vi "Autonomous Independent.vi"   [LabVIEW 2013]
doc: "This VI is called when autonomous begins, and will automatically be terminated when autonomous ends. You can carry out timed or sensor driven robot movement independently without needing to return to the caller."
uses:
  <vilib>/Rock Robotics/WPI/Solenoid/WPI_SolenoidValue.ctl
  Robot Global Data.vi
  <vilib>/Rock Robotics/WPI/RobotDrive/WPI_RobotDriveGetSetRefNum.vi
  <vilib>/Rock Robotics/WPI/RobotDrive/WPI_RobotDriveArcadeDrive_Standard(NoSaturation).vi
  <vilib>/Rock Robotics/WPI/Solenoid/WPI_SolenoidSetEnum.vi
panel:
  # "Be sure to right-click and choose Data Operations>>Make Current Value default if you want to save the array values with the VI"
types:
  T1 = typedef "WPI_RobotDriveDevRef.ctl" = cluster{"DevStatus":errorcluster, "Motors[]":T2[], "Square Inputs":bool, "Max Output":dbl, "Isochronous":bool}
  T2 = typedef "WPI_MotorControlDeviceRef.ctl" = cluster{"DeviceStatus":errorcluster, "Type":enum16{"PWM", "CAN"}, "PWM":cluster{"Digital Module":T3, "PWM Channel":T4, "DeadBand":T5}, "CAN":cluster{"Device Number":u8, "Control Mode":T6, "Semaphore":T7, "Max Vout":dbl}, "Invert":bool, "TransformRef":T8, "InvTransformRef":T8}
  T3 = typedef "FPGA_TypedefDigitalModule.ctl" = enum16{"Digital Module 1", "Digital Module 2"}
  T4 = typedef "FPGA_DIOPWMChannel.ctl" = enum8{"PWM 1", "PWM 2", "PWM 3", "PWM 4", "PWM 5", "PWM 6", "PWM 7", "PWM 8", "PWM 9", "PWM 10", "Invalid"}
  T5 = typedef "WPI_PWMDeadband.ctl" = cluster{"Name":string, "maxPositivePwm":i32, "minPositivePwm":i32, "centerPwm":i32, "maxNegativePwm":i32, "minNegativePwm":i32, "angularRange":u16}
  T6 = typedef "WPI_CANJaguar_ControlMode.ctl" = enum8{"Percent VBus", "Current", "Speed", "Position", "Voltage"}
  T7 = typedef "Semaphore RefNum" = refnum<k1>
  T8 = typedef "WPI_PWMTransform_ConPane.ctl" = refnum<vi>
  T9 = typedef "WPI_SolenoidValue.ctl" = enum16{"Off", "On", "Forward", "Reverse"}
  T10 = typedef "WPI_DigitalInputDevRef.ctl" = cluster{"DevStatus":errorcluster, "DIO Channel":T11, "Digital Module":T3}
  T11 = typedef "FPGA_DIOChannel.ctl" = enum8{"DIO 1", "DIO 2", "DIO 3", "DIO 4", "DIO 5", "DIO 6", "DIO 7", "DIO 8", "DIO 9", "DIO 10", "DIO 11", "DIO 12", "DIO 13", "DIO 14", "Invalid"}
  T12 = typedef "WPI_SolenoidDevRef.ctl" = cluster{"DevStatus":errorcluster, "Solenoid Module":T13, "Forward Solenoid Channel":T14, "Reverse Solenoid Channel":T14}
  T13 = typedef "FPGA_TypedefSolenoidModule.ctl" = enum16{"Solenoid Module 1", "Solenoid Module 2"}
  T14 = typedef "WPI_SolenoidChannel.ctl" = enum8{"Solenoid 1", "Solenoid 2", "Solenoid 3", "Solenoid 4", "Solenoid 5", "Solenoid 6", "Solenoid 7", "Solenoid 8", "Invalid"}
  T15 = typedef "WPI_AnalogChannelDevRef.ctl" = cluster{"DevStatus":errorcluster, "Analog Module":T16, "Analog Channel":T17}
  T16 = typedef "FPGA_TypedefAnalogModule.ctl" = enum16{"Analog Module 1", "Analog Module 2"}
  T17 = typedef "FPGA_AIChannel.ctl" = enum8{"AI 1", "AI 2", "AI 3", "AI 4", "AI 5", "AI 6", "AI 7", "AI 8", "Invalid"}
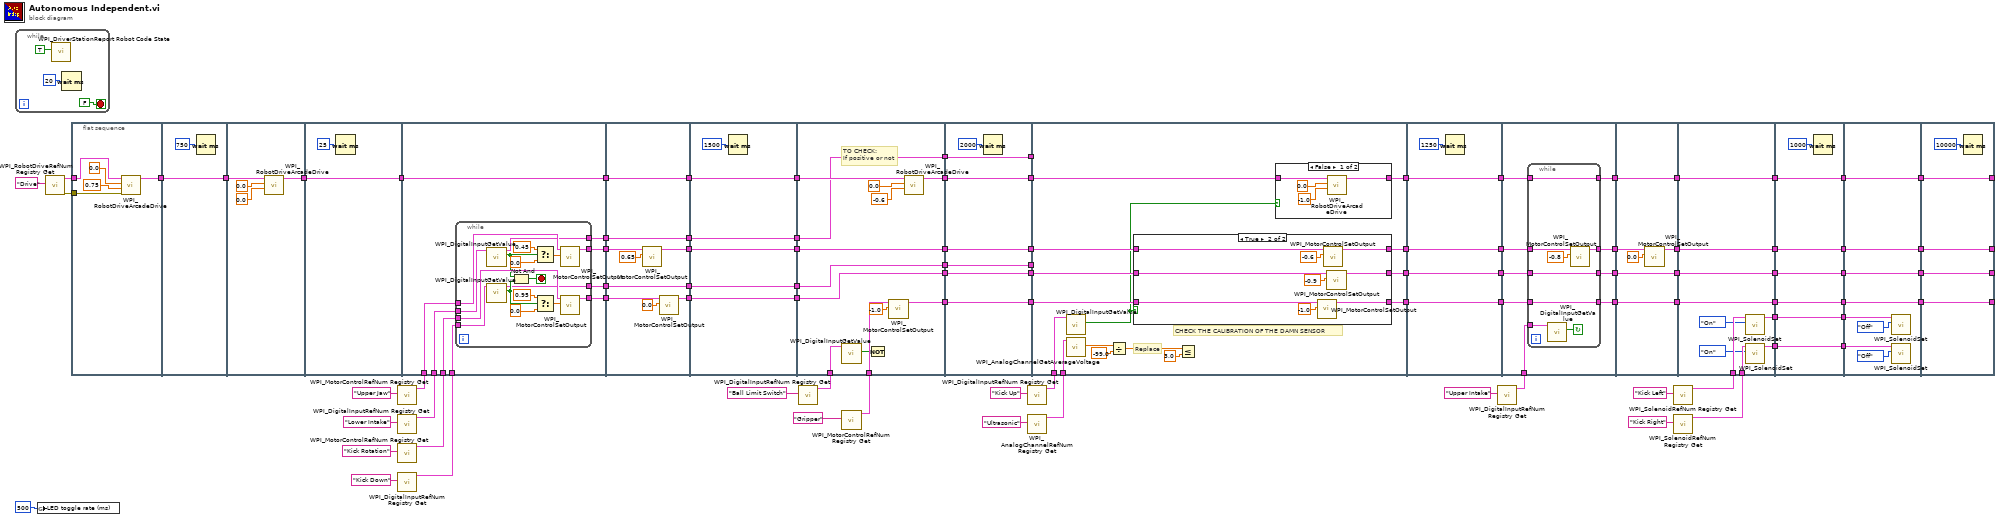
[diagram p0: block diagram]
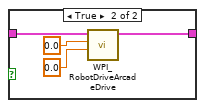
[diagram p2: hidden frame]
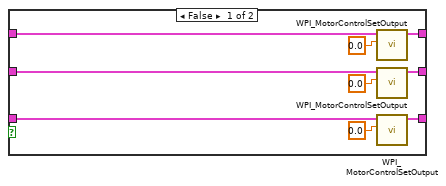
[diagram p3: hidden frame]
diagram:
  n1 = while {
    stop <- FALSE stop-if-true
    n2 = call <vilib>:"WPI_DriverStationReport Robot Code State.vi"("Autonomous"=TRUE) -> ()  [unwired: 10 in, 1 out]
    n3 = Wait (ms)(milliseconds to wait=u32 20) -> ()  [unwired: 1 out]
  }
  n4 = global write "Robot Global Data.vi" "LED toggle rate (ms)"(u32 500 ("LED ms toggle rate")) -> ()
  n5 = call <vilib>:"WPI_RobotDriveRefNum Registry Get.vi"("refnum name"="Drive") -> ("error out"=w84:errorcluster, "RobotDriveDevRef"=w85:T1)  [unwired: 9 in]
  n6 = flat-sequence {
    tunnel: w85 -> [w95]
    tunnel: w84 -> [w94]
    tunnel: [w93] -> w73
    tunnel: w73 -> [w99]
    tunnel: [w99] -> w72
    tunnel: [w102] -> w71
    tunnel: w72 -> [w103]
    tunnel: w71 -> [w105]
    tunnel: [w105] -> w70
    tunnel: w83 -> [w113]
    tunnel: w81 -> [w110]
    tunnel: w78 -> [w114]
    tunnel: [w112] -> w77
    tunnel: w70 -> [w112]
    tunnel: w76 -> [w111]
    tunnel: [w109] -> w75
    tunnel: [w108] -> w74
    tunnel: [w107] -> w69
    tunnel: [w106] -> w68
    tunnel: w77 -> [w136]
    tunnel: w75 -> [w139]
    tunnel: w74 -> [w140]
    tunnel: w69 -> [w133]
    tunnel: w68 -> [w135]
    tunnel: [w136] -> w10
    tunnel: [w135] -> w8
    tunnel: [w134] -> w6
    tunnel: [w133] -> w4
    tunnel: [w132] -> w2
    tunnel: w10 -> [w146]
    tunnel: [w146] -> w9
    tunnel: w8 -> [w145]
    tunnel: [w145] -> w7
    tunnel: w6 -> [w144]
    tunnel: [w144] -> w5
    tunnel: w4 -> [w143]
    tunnel: [w143] -> w3
    tunnel: w2 -> [w142]
    tunnel: [w142] -> w1
    tunnel: w9 -> [w159]
    tunnel: w67 -> [w158]
    tunnel: [w157] -> w22
    tunnel: [w156] -> w20
    tunnel: w65 -> [w155]
    tunnel: [w154] -> w18
    tunnel: w7 -> [w154]
    tunnel: [w153] -> w16
    tunnel: w5 -> [w153]
    tunnel: [w152] -> w14
    tunnel: w3 -> [w152]
    tunnel: [w151] -> w12
    tunnel: w1 -> [w151]
    tunnel: w22 -> [w166]
    tunnel: [w166] -> w21
    tunnel: w20 -> [w165]
    tunnel: [w165] -> w19
    tunnel: w18 -> [w164]
    tunnel: [w164] -> w17
    tunnel: w16 -> [w163]
    tunnel: [w163] -> w15
    tunnel: w14 -> [w162]
    tunnel: [w162] -> w13
    tunnel: w12 -> [w161]
    tunnel: [w161] -> w11
    tunnel: w21 -> [w181]
    tunnel: w19 -> [w178]
    tunnel: w17 -> [_]
    tunnel: w15 -> [w179]
    tunnel: w13 -> [_]
    tunnel: w11 -> [w177]
    tunnel: w63 -> [w180]
    tunnel: w61 -> [w176]
    tunnel: [w175] -> w30
    tunnel: [w174] -> w28
    tunnel: [w173] -> w26
    tunnel: [w172] -> w24
    tunnel: w30 -> [w212]
    tunnel: [w212] -> w29
    tunnel: w28 -> [w211]
    tunnel: [w211] -> w27
    tunnel: w26 -> [w210]
    tunnel: [w210] -> w25
    tunnel: w24 -> [w209]
    tunnel: [w209] -> w23
    tunnel: w29 -> [w221]
    tunnel: w27 -> [w219]
    tunnel: w59 -> [w218]
    tunnel: w25 -> [w215]
    tunnel: w23 -> [w213]
    tunnel: [w220] -> w58
    tunnel: [w217] -> w57
    tunnel: [w216] -> w56
    tunnel: [w214] -> w55
    tunnel: w58 -> [w235]
    tunnel: w57 -> [w232]
    tunnel: w56 -> [w234]
    tunnel: w55 -> [w233]
    tunnel: [w235] -> w54
    tunnel: [w234] -> w53
    tunnel: [w233] -> w52
    tunnel: [w230] -> w51
    tunnel: w54 -> [w245]
    tunnel: w53 -> [w244]
    tunnel: w52 -> [w243]
    tunnel: w51 -> [w242]
    tunnel: w48 -> [w241]
    tunnel: w47 -> [w240]
    tunnel: [w245] -> w46
    tunnel: [w244] -> w44
    tunnel: [w243] -> w42
    tunnel: [w242] -> w40
    tunnel: [w237] -> w38
    tunnel: [w236] -> w36
    tunnel: w46 -> [w252]
    tunnel: [w252] -> w45
    tunnel: w44 -> [w251]
    tunnel: [w251] -> w43
    tunnel: w42 -> [w250]
    tunnel: [w250] -> w41
    tunnel: w40 -> [w249]
    tunnel: [w249] -> w39
    tunnel: w38 -> [w248]
    tunnel: [w248] -> w37
    tunnel: w36 -> [w247]
    tunnel: [w247] -> w35
    tunnel: w45 -> [w260]
    tunnel: w43 -> [w259]
    tunnel: w41 -> [w258]
    tunnel: w39 -> [w257]
    tunnel: w37 -> [w255]
    tunnel: w35 -> [w256]
    tunnel: [w260] -> w34
    tunnel: [w259] -> w33
    tunnel: [w258] -> w32
    tunnel: [w257] -> w31
    tunnel: [w262] -> _
    tunnel: [w263] -> _
    tunnel: [w264] -> _
    tunnel: [w265] -> _
    tunnel: w34 -> [w265]
    tunnel: w33 -> [w264]
    tunnel: w32 -> [w263]
    tunnel: w31 -> [w262]
    frame #0 {
      n7 = call-poly <vilib>:"WPI_RobotDriveArcadeDrive.vi"("error in (no error)"=w94, "Y axis value"=0.75, "X axis value"=0.0, "RobotDriveDevRef"=w95) -> ("RobotDriveDevRef"=w93:T1)  [unwired: 5 in, 2 out]
    }
    frame #1 {
      n8 = Wait (ms)(milliseconds to wait=u32 750) -> ()  [unwired: 1 out]
    }
    frame #2 {
      n9 = call-poly <vilib>:"WPI_RobotDriveArcadeDrive.vi"("Y axis value"=0.0, "X axis value"=0.0, "RobotDriveDevRef"=w103) -> ("RobotDriveDevRef"=w102:T1)  [unwired: 6 in, 2 out]
    }
    frame #3 {
      n10 = Wait (ms)(milliseconds to wait=u32 25) -> ()  [unwired: 1 out]
    }
    frame #4 {
      n11 = while {
        tunnel: w114 -> [w127]
        tunnel: w113 -> [w125]
        tunnel: w111 -> [w123]
        tunnel: w110 -> [w122]
        tunnel: [w119] -> w109
        tunnel: [w118] -> w108
        tunnel: [w117] -> w107
        tunnel: [w116] -> w106
        stop <- w124 stop-if-true
        n12 = call <vilib>:"WPI_DigitalInputGetValue.vi"("DigitalInputDevRef"=w127) -> ("Value"=w115:bool, "DigitalInputDevRef"=w116:T10)  [unwired: 8 in, 1 out]
        n13 = call <vilib>:"WPI_DigitalInputGetValue.vi"("DigitalInputDevRef"=w123) -> ("Value"=w120:bool, "DigitalInputDevRef"=w117:T10)  [unwired: 8 in, 1 out]
        n14 = Not And(1:w120, 2:w115) -> (0:w124:bool)
        n15 = Select(t=0.45, s=w115, f=0.0) -> (s? t:f=w126:dbl)
        n16 = Select(t=0.95, s=w120, f=0.0) -> (s? t:f=w121:dbl)
        n17 = call <vilib>:"WPI_MotorControlSetOutput.vi"("Output"=w126, "MotorControlDevRef"=w125) -> ("MotorControlDevRef"=w119:T2)  [unwired: 7 in, 2 out]
        n18 = call <vilib>:"WPI_MotorControlSetOutput.vi"("Output"=w121, "MotorControlDevRef"=w122) -> ("MotorControlDevRef"=w118:T2)  [unwired: 7 in, 2 out]
      }
    }
    frame #5 {
      n19 = call <vilib>:"WPI_MotorControlSetOutput.vi"("Output"=0.65, "MotorControlDevRef"=w139) -> ("MotorControlDevRef"=w134:T2)  [unwired: 7 in, 2 out]
      n20 = call <vilib>:"WPI_MotorControlSetOutput.vi"("Output"=0.0, "MotorControlDevRef"=w140) -> ("MotorControlDevRef"=w132:T2)  [unwired: 7 in, 2 out]
    }
    frame #6 {
      n21 = Wait (ms)(milliseconds to wait=u32 1500) -> ()  [unwired: 1 out]
    }
    frame #7 {
      # "TO CHECK:\nIf positive or not"
      n22 = call <vilib>:"WPI_DigitalInputGetValue.vi"("DigitalInputDevRef"=w155) -> ("Value"=w147:bool)  [unwired: 8 in, 2 out]
      n23 = Not(x=w147) -> ()  [unwired: 1 out]
      n24 = call <vilib>:"WPI_MotorControlSetOutput.vi"("Output"=-1.0, "MotorControlDevRef"=w158) -> ("MotorControlDevRef"=w156:T2)  [unwired: 7 in, 2 out]
      n25 = call-poly <vilib>:"WPI_RobotDriveArcadeDrive.vi"("Y axis value"=-0.6, "X axis value"=0.0, "RobotDriveDevRef"=w159) -> ("RobotDriveDevRef"=w157:T1)  [unwired: 6 in, 2 out]
    }
    frame #8 {
      n26 = Wait (ms)(milliseconds to wait=u32 2000) -> ()  [unwired: 1 out]
    }
    frame #9 {
      # "CHECK THE CALIBRATION OF THE DAMN SENSOR"
      # "Replace"
      n27 = call <vilib>:"WPI_DigitalInputGetValue.vi"("DigitalInputDevRef"=w180) -> ("Value"=w167:bool)  [unwired: 8 in, 2 out]
      n28 = call <vilib>:"WPI_AnalogChannelGetAverageVoltage.vi"("AIDeviceRef"=w176) -> ("Voltage"=w170:dbl)  [unwired: 8 in, 2 out]
      n29 = Divide(x=w170, y=-99.0) -> (x/y=w169:dbl)
      n30 = case shown="True" w167 {
        tunnel: w178 -> [w197 w207]
        tunnel: w177 -> [w196 w204]
        tunnel: w179 -> [w193 w203]
        tunnel: [w192 w201] -> w174
        tunnel: [w190 w200] -> w173
        tunnel: [w191 w199] -> w172
        frame False {
          n31 = call <vilib>:"WPI_MotorControlSetOutput.vi"("Output"=0.0, "MotorControlDevRef"=w193) -> ("MotorControlDevRef"=w192:T2)  [unwired: 7 in, 2 out]
          n32 = call <vilib>:"WPI_MotorControlSetOutput.vi"("Output"=0.0, "MotorControlDevRef"=w196) -> ("MotorControlDevRef"=w191:T2)  [unwired: 7 in, 2 out]
          n33 = call <vilib>:"WPI_MotorControlSetOutput.vi"("Output"=0.0, "MotorControlDevRef"=w197) -> ("MotorControlDevRef"=w190:T2)  [unwired: 7 in, 2 out]
        }
        frame True {
          n34 = call <vilib>:"WPI_MotorControlSetOutput.vi"("Output"=-1.0, "MotorControlDevRef"=w207) -> ("MotorControlDevRef"=w200:T2)  [unwired: 7 in, 2 out]
          n35 = call <vilib>:"WPI_MotorControlSetOutput.vi"("Output"=-0.6, "MotorControlDevRef"=w203) -> ("MotorControlDevRef"=w201:T2)  [unwired: 7 in, 2 out]
          n36 = call <vilib>:"WPI_MotorControlSetOutput.vi"("Output"=-0.9, "MotorControlDevRef"=w204) -> ("MotorControlDevRef"=w199:T2)  [unwired: 7 in, 2 out]
        }
      }
      n37 = Less Or Equal?(x=w169, y=3.0) -> ()  [unwired: 1 out]
      n38 = case shown="False" w167 {
        tunnel: w181 -> [w183 w187]
        tunnel: [w182 w186] -> w175
        frame False {
          n39 = call-poly <vilib>:"WPI_RobotDriveArcadeDrive.vi"("Y axis value"=-1.0, "X axis value"=0.0, "RobotDriveDevRef"=w183) -> ("RobotDriveDevRef"=w182:T1)  [unwired: 6 in, 2 out]
        }
        frame True {
          n40 = call-poly <vilib>:"WPI_RobotDriveArcadeDrive.vi"("Y axis value"=0.0, "X axis value"=0.0, "RobotDriveDevRef"=w187) -> ("RobotDriveDevRef"=w186:T1)  [unwired: 6 in, 2 out]
        }
      }
    }
    frame #10 {
      n41 = Wait (ms)(milliseconds to wait=u32 1250) -> ()  [unwired: 1 out]
    }
    frame #11 {
      n42 = while {
        tunnel: w221 -> [w229]
        tunnel: [w229] -> w220
        tunnel: w219 -> [w227]
        tunnel: w218 -> [w226]
        tunnel: [w224] -> w217
        tunnel: [w223] -> w216
        tunnel: w215 -> [w223]
        tunnel: [w222] -> w214
        tunnel: w213 -> [w222]
        stop <- w225 continue-if-true
        n43 = call <vilib>:"WPI_DigitalInputGetValue.vi"("DigitalInputDevRef"=w226) -> ("Value"=w225:bool)  [unwired: 8 in, 2 out]
        n44 = call <vilib>:"WPI_MotorControlSetOutput.vi"("Output"=-0.8, "MotorControlDevRef"=w227) -> ("MotorControlDevRef"=w224:T2)  [unwired: 7 in, 2 out]
      }
    }
    frame #12 {
      n45 = call <vilib>:"WPI_MotorControlSetOutput.vi"("Output"=0.0, "MotorControlDevRef"=w232) -> ("MotorControlDevRef"=w230:T2)  [unwired: 7 in, 2 out]
    }
    frame #13 {
      n46 = call-poly <vilib>:"WPI_SolenoidSet.vi"("Value"=WPI_SolenoidValue."On", "SolenoidDevRef"=w240) -> ("SolenoidDevRef"=w237:T12)  [unwired: 8 in, 1 out]
      n47 = call-poly <vilib>:"WPI_SolenoidSet.vi"("Value"=WPI_SolenoidValue."On", "SolenoidDevRef"=w241) -> ("SolenoidDevRef"=w236:T12)  [unwired: 8 in, 1 out]
    }
    frame #14 {
      n48 = Wait (ms)(milliseconds to wait=u32 1000) -> ()  [unwired: 1 out]
    }
    frame #15 {
      n49 = call-poly <vilib>:"WPI_SolenoidSet.vi"("Value"=WPI_SolenoidValue."Off", "SolenoidDevRef"=w255) -> ()  [unwired: 8 in, 2 out]
      n50 = call-poly <vilib>:"WPI_SolenoidSet.vi"("Value"=WPI_SolenoidValue."Off", "SolenoidDevRef"=w256) -> ()  [unwired: 8 in, 2 out]
    }
    frame #16 {
      n51 = Wait (ms)(milliseconds to wait=u32 10000) -> ()  [unwired: 1 out]
    }
  }
  n52 = call <vilib>:"WPI_MotorControlRefNum Registry Get.vi"("refnum name"="Upper Jaw") -> ("MotorControlDevRef"=w83:T2)  [unwired: 9 in, 1 out]
  n53 = call <vilib>:"WPI_DigitalInputRefNum Registry Get.vi"("refnum name"="Lower Intake") -> ("DigitalInputDevRef"=w78:T10)  [unwired: 9 in, 1 out]
  n54 = call <vilib>:"WPI_MotorControlRefNum Registry Get.vi"("refnum name"="Kick Rotation") -> ("MotorControlDevRef"=w81:T2)  [unwired: 9 in, 1 out]
  n55 = call <vilib>:"WPI_DigitalInputRefNum Registry Get.vi"("refnum name"="Kick Down") -> ("DigitalInputDevRef"=w76:T10)  [unwired: 9 in, 1 out]
  n56 = call <vilib>:"WPI_DigitalInputRefNum Registry Get.vi"("refnum name"="Ball Limit Switch") -> ("DigitalInputDevRef"=w65:T10)  [unwired: 9 in, 1 out]
  n57 = call <vilib>:"WPI_MotorControlRefNum Registry Get.vi"("refnum name"="Gripper") -> ("MotorControlDevRef"=w67:T2)  [unwired: 9 in, 1 out]
  n58 = call <vilib>:"WPI_DigitalInputRefNum Registry Get.vi"("refnum name"="Kick Up") -> ("DigitalInputDevRef"=w63:T10)  [unwired: 9 in, 1 out]
  n59 = call <vilib>:"WPI_AnalogChannelRefNum Registry Get.vi"("refnum name"="Ultrasonic") -> ("AIDeviceRef"=w61:T15)  [unwired: 9 in, 1 out]
  n60 = call <vilib>:"WPI_DigitalInputRefNum Registry Get.vi"("refnum name"="Upper Intake") -> ("DigitalInputDevRef"=w59:T10)  [unwired: 9 in, 1 out]
  n61 = call <vilib>:"WPI_SolenoidRefNum Registry Get.vi"("refnum name"="Kick Left") -> ("SolenoidDevRef"=w47:T12)  [unwired: 9 in, 1 out]
  n62 = call <vilib>:"WPI_SolenoidRefNum Registry Get.vi"("refnum name"="Kick Right") -> ("SolenoidDevRef"=w48:T12)  [unwired: 9 in, 1 out]
